vi "GetDigitizerDataV1729A.vi"(8 "error in (no error)":errorcluster, 10 "handle in":i32, 11 "VME Base Address":u32) -> (0 "error out":errorcluster, 1 "handle out":i32, 2 "Waveform":u32[](array[numeric]), 3 "TRIG_REC":u32)   [LabVIEW 2014]
uses:
  Program Files (x86)/CAEN/Comm/labview/CAENComm.lvlib
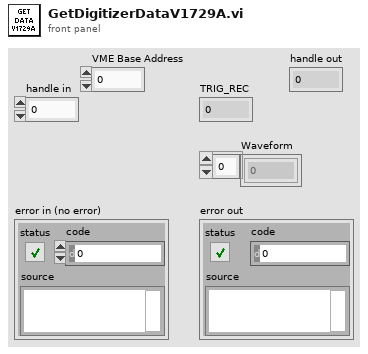
[diagram p1: front panel]
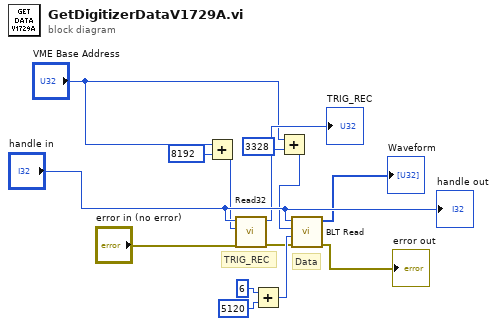
[diagram p0: block diagram]
diagram:
  # "Data"
  # "TRIG_REC"
  n1 = Add(x="VME Base Address", y=u32 8192 ("x")) -> (x+y=w3:u32)
  n2 = call "Read32.vi"("error in (no error)"="error in (no error)", "Address"=w3, "handle"="handle in") -> ("error out"=w6:errorcluster, "Data"=→"TRIG_REC":u32)  [unwired: 7 in]
  n3 = Add(x=6 ("BltSize"), y=5120 ("BltSize")) -> (x+y=w10:i32)
  n4 = Add(x="VME Base Address", y=u32 3328 ("x")) -> (x+y=w7:u32)
  n5 = call "BLT Read.vi"("error in (no error)"=w6, "BltSize"=w10, "Address"=w7, "handle"="handle in") -> ("error out"=→"error out":errorcluster, "Buff"=→"Waveform":u32[])  [unwired: 5 in, 1 out]
  "handle out" <- "handle in"
